vi "TDC001_motor_control tw.vi"(8 "Move":bool, 10 "Moving parameters":T1={"Velocity (mm/s)"=0.5, "Abs position (mm)"=0.0, "Lasting time (s)"=20.0}, 11 "Serial":i32=83858441) -> (3 "pfPosition (mm)":sgl)   [LabVIEW 2015]
panel:
  out "error out":errorcluster
  in  "Home (for the calibration)":bool
  in  "MG17Motor":refnum<k7>(container)
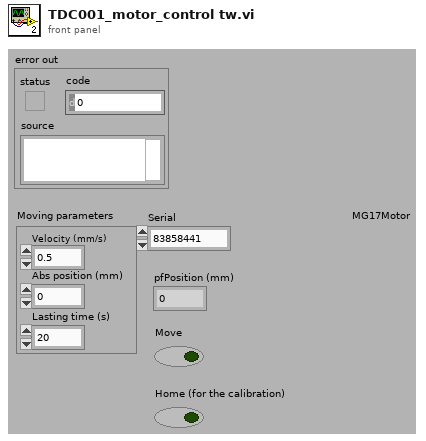
[diagram p1: front panel]
types:
  T1 = cluster{"Velocity (mm/s)":dbl, "Abs position (mm)":dbl, "Lasting time (s)":dbl}
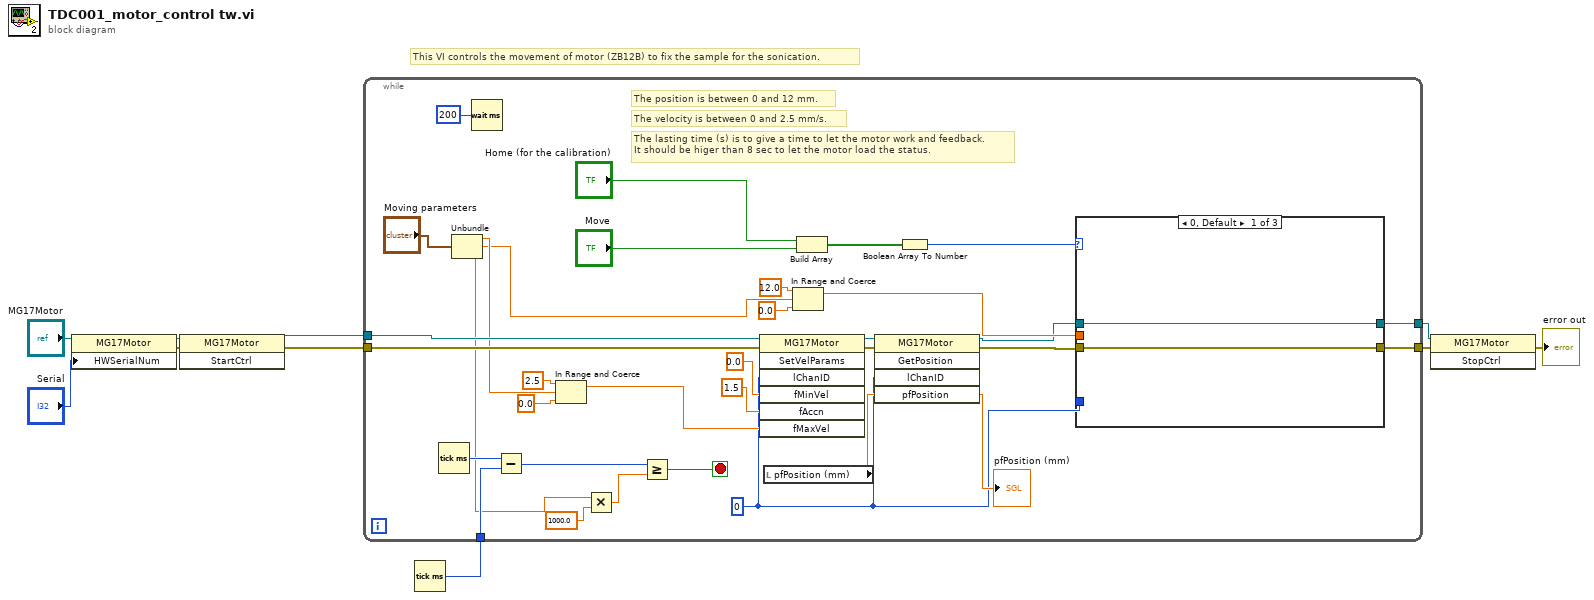
[diagram p0: block diagram]
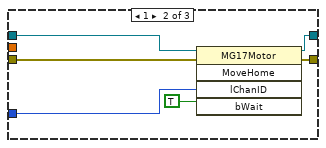
[diagram p2: hidden frame]
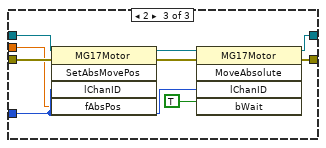
[diagram p3: hidden frame]
diagram:
  # "This VI controls the movement of motor (ZB12B) to fix the sample for the sonication."
  n1 = property class="MG17Motor"(reference="MG17Motor", "HWSerialNum"="Serial") -> (reference out=w8:refnum<k7>, error out=w7:errorcluster)  [unwired: 1 in]
  n2 = invoke class="MG17Motor" method="StartCtrl"(reference=w8, error in=w7) -> (reference out=w2:refnum<k7>, error out=w1:errorcluster)  [unwired: 1 in, 1 out]
  n3 = Tick Count (ms)() -> (millisecond timer value=w3:u32)
  n4 = while {
    tunnel: w2 -> [w32]
    tunnel: [w38] -> w4
    tunnel: w1 -> [w30]
    tunnel: [w37] -> w6
    tunnel: w3 -> [w15]
    stop <- w18 stop-if-true
    w23 = 0 ("lChanID")
    # "The lasting time (s) is to give a time to let the motor work and feedback.\nIt should be higer than 8 sec to let the motor load the status."
    # "The velocity is between 0 and 2.5 mm/s."
    # "The position is between 0 and 12 mm."
    n5 = Tick Count (ms)() -> (millisecond timer value=w20:u32)
    n6 = Unbundle("Moving parameters") -> ("Velocity (mm/s)"=w13:dbl, "Abs position (mm)"=w12:dbl, "Lasting time (s)"=w11:dbl)
    n7 = Wait (ms)(milliseconds to wait=u32 200) -> ()  [unwired: 1 out]
    n8 = Subtract(x=w20, y=w15) -> (x-y=w17:u32)
    n9 = In Range and Coerce(upper limit=2.5, x=w13, lower limit=0.0) -> (coerced(x)=w26:dbl)  [unwired: 1 out]
    n10 = Multiply(x=w11, y=1000.0) -> (x*y=w19:dbl)
    n11 = Greater Or Equal?(x=w17, y=w19) -> (x >= y?=w18:bool)
    n12 = invoke class="MG17Motor" method="SetVelParams"(reference=w32, error in=w30, "lChanID"=w23, "fMinVel"=sgl 0.0, "fAccn"=sgl 1.5, "fMaxVel"=w26) -> (reference out=w31:refnum<k7>, error out=w29:errorcluster)  [unwired: 1 in, 5 out]
    n13 = local read "pfPosition (mm)"() -> (w42:sgl)
    n14 = In Range and Coerce(upper limit=12.0, x=w12, lower limit=0.0) -> (coerced(x)=w35:dbl)  [unwired: 1 out]
    n15 = Build Array("Home (for the calibration)", "Move") -> (w40:bool[])
    n16 = invoke class="MG17Motor" method="GetPosition"(reference=w31, error in=w29, "lChanID"=w23, "pfPosition"=w42) -> (reference out=w21:refnum<k7>, error out=w22:errorcluster, "pfPosition"=→"pfPosition (mm)":sgl)  [unwired: 1 in, 2 out]
    n17 = Boolean Array To Number(Boolean array=w40) -> (number=w39:u32)
    n18 = case shown="0, Default" w39 {
      tunnel: w21 -> [w46 w52 w61]
      tunnel: w22 -> [w45 w50 w60]
      tunnel: [w46 w51 w56] -> w38
      tunnel: [w45 w49 w55] -> w37
      tunnel: w23 -> [_ w48 w58]
      tunnel: w35 -> [_ _ w53]
      frame 0, Default {
      }
      frame 1 {
        n19 = invoke class="MG17Motor" method="MoveHome"(reference=w52, error in=w50, "lChanID"=w48, "bWait"=TRUE) -> (reference out=w51:refnum<k7>, error out=w49:errorcluster)  [unwired: 1 in, 3 out]
      }
      frame 2 {
        n20 = invoke class="MG17Motor" method="SetAbsMovePos"(reference=w61, error in=w60, "lChanID"=w58, "fAbsPos"=w53) -> (reference out=w59:refnum<k7>, error out=w57:errorcluster)  [unwired: 1 in, 3 out]
        n21 = invoke class="MG17Motor" method="MoveAbsolute"(reference=w59, error in=w57, "lChanID"=w58, "bWait"=TRUE) -> (reference out=w56:refnum<k7>, error out=w55:errorcluster)  [unwired: 1 in, 3 out]
      }
    }
  }
  n22 = invoke class="MG17Motor" method="StopCtrl"(reference=w4, error in=w6) -> (error out=→"error out":errorcluster)  [unwired: 1 in, 2 out]
